vi "ROI_to_INP.vi"(8 "error in (no error)":errorcluster, 9 "Show Message":bool, 10 "ROI Values":T1) -> (0 "error out":errorcluster)   [LabVIEW 2015]
uses:
  <vilib>/Utility/config.llb/Write Key (String).vi
  <vilib>/Utility/config.llb/Write Key (I32).vi
  <vilib>/Utility/config.llb/NI_LVConfig.lvlib
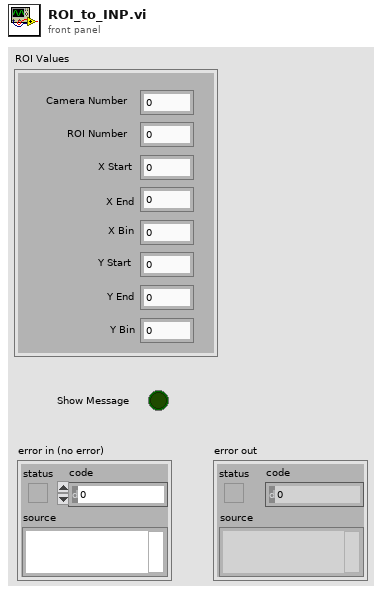
[diagram p1: front panel]
types:
  T1 = cluster{"Camera Number":i32, "ROI Number":i32, "X Start":i32, "X End":i32, "X Bin":i32, "Y Start":i32, "Y End":i32, "Y Bin":i32}
  T2 = typedef "NI_LVConfig.lvlib/Config Data RefNum.ctl" = refnum<k1>
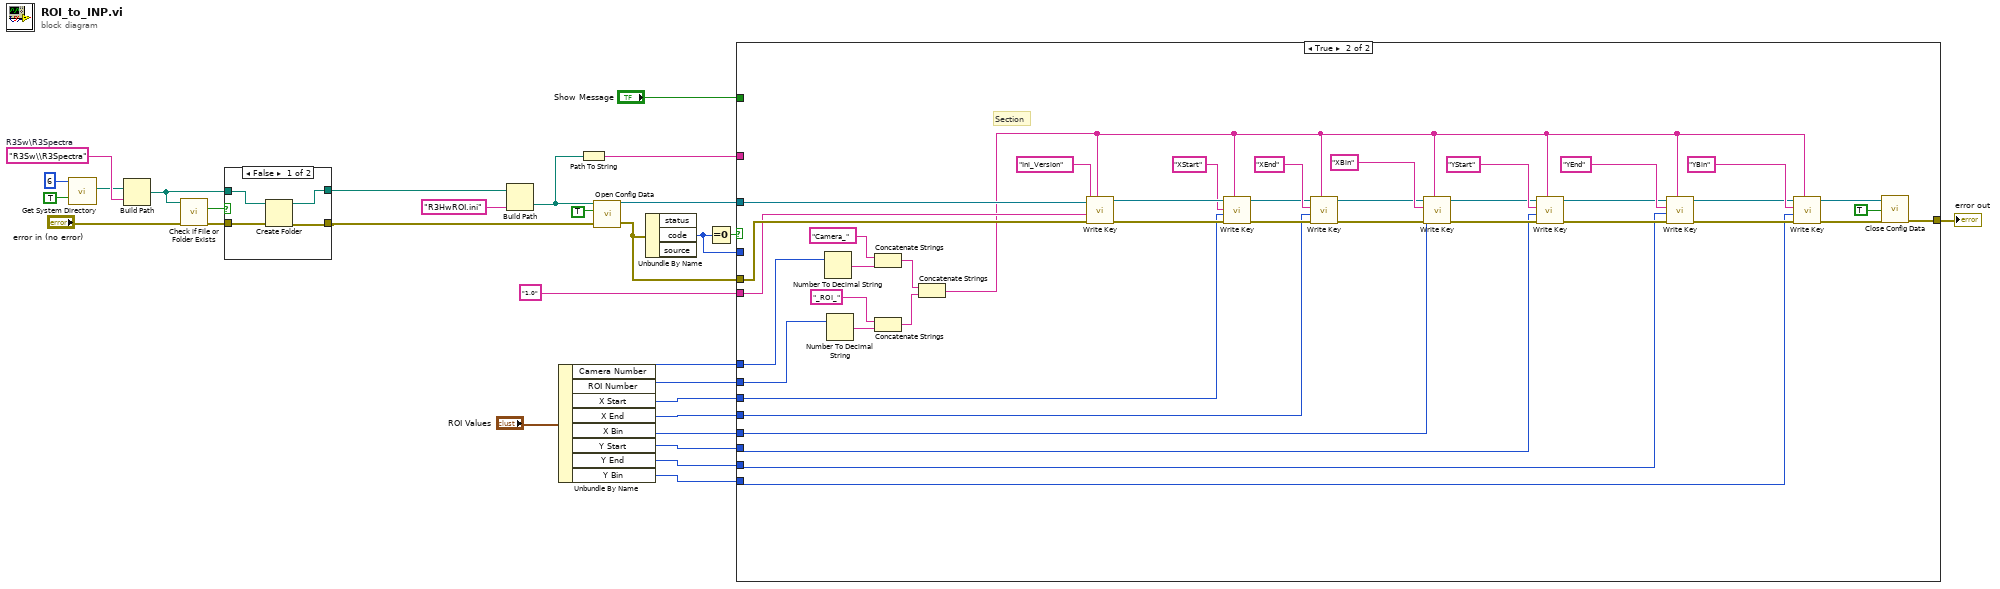
[diagram p0: block diagram]
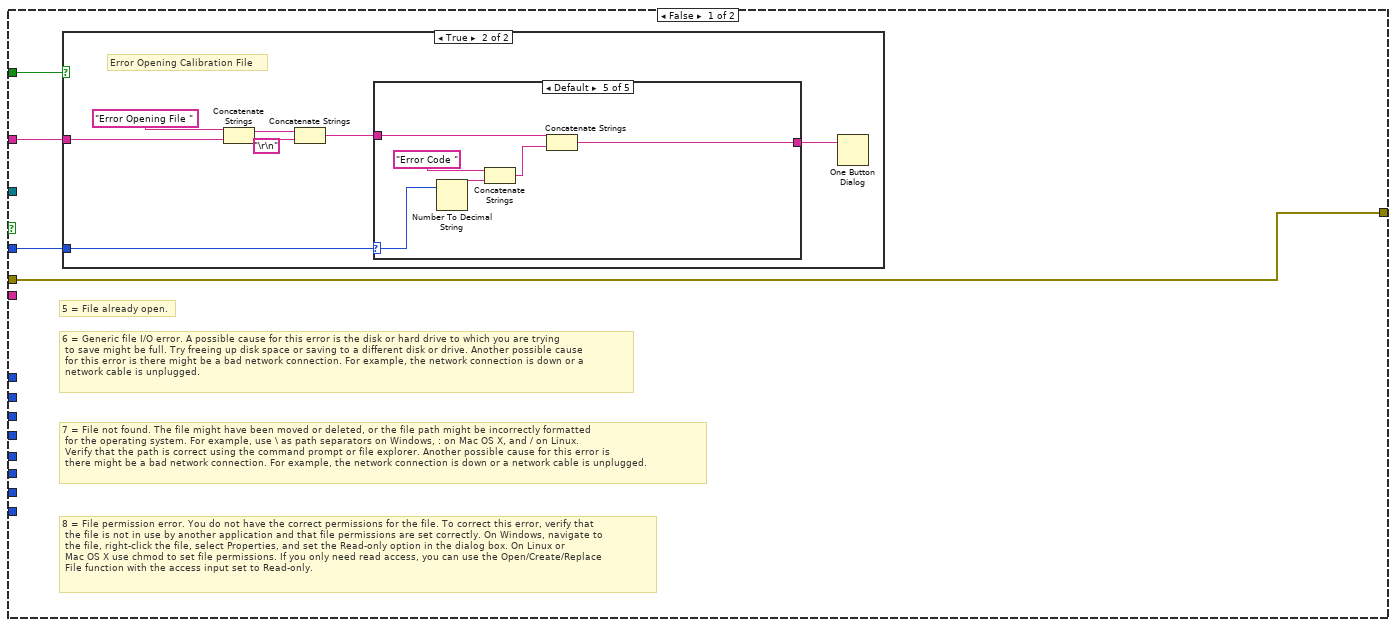
[diagram p3: hidden frame]
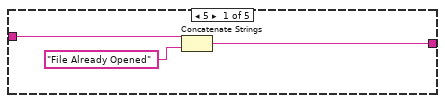
[diagram p5: hidden frame]
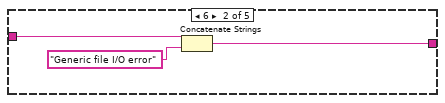
[diagram p6: hidden frame]
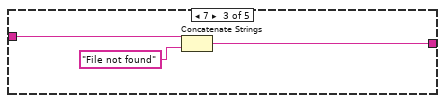
[diagram p7: hidden frame]
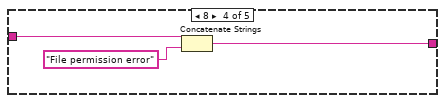
[diagram p8: hidden frame]
diagram:
  w6 = "R3Sw\\R3Spectra"  # R3Sw\R3Spectra
  n1 = call <vilib>:"Get System Directory.vi"("create directory if not found? (F)"=TRUE, "system directory type"=6) -> ("system directory"=w5:path)  [unwired: 9 in]
  n2 = Build Path(base path=w5, name or relative path=w6) -> (appended path=w4:path)
  n3 = call <vilib>:"Check if File or Folder Exists.vi"("error in (no error)"="error in (no error)", "path"=w4) -> ("error out"=w9:errorcluster, "file or folder exists?"=w10:bool)  [unwired: 7 in, 1 out]
  n4 = case shown="False" w10 {
    tunnel: w9 -> [w32 w35]
    tunnel: [w31 w35] -> w2
    tunnel: w4 -> [w33 w34]
    tunnel: [w30 w34] -> w1
    frame False {
      n5 = Create Folder(path (use dialog)=w33, error in=w32) -> (created path=w30:path, error out=w31:errorcluster)  [unwired: 1 in, 1 out]
    }
    frame True {
    }
  }
  n6 = Build Path(base path=w1, name or relative path="R3HwROI.ini") -> (appended path=w16:path)
  n7 = Unbundle By Name("ROI Values") -> ("Camera Number"=w12:i32, "X Start"=w13:i32, "X End"=w22:i32, "X Bin"=w21:i32, "Y Start"=w20:i32, "Y End"=w19:i32, "Y Bin"=w18:i32)  [unwired: 1 out]
  n8 = Path To String(path=w16) -> (string=w15:string)
  n9 = call <vilib>:"Open Config Data.vi"("error in (no error)"=w2, "create file if necessary (T)"=TRUE, "configuration file path"=w16) -> ("error out"=w26:errorcluster, "refnum"=w27:T2)  [unwired: 6 in, 1 out]
  n10 = Unbundle By Name(w26) -> ("code"=w25:i32)  [unwired: 2 out]
  n11 = Equal To 0?(x=w25) -> (x = 0?=w28:bool)
  n12 = case shown="True" w28 {
    tunnel: w27 -> [_ w104]
    tunnel: w26 -> [w37 w103]
    tunnel: w25 -> [w38 _]
    tunnel: w15 -> [w39 _]
    tunnel: [w37 w102] -> w24
    tunnel: w12 -> [_ w100]
    tunnel: "1.0" -> [_ w101]
    tunnel: w13 -> [_ w73]
    tunnel: w22 -> [_ w71]
    tunnel: w21 -> [_ w72]
    tunnel: w20 -> [_ w68]
    tunnel: w19 -> [_ w70]
    tunnel: w18 -> [_ w69]
    tunnel: w12 -> [_ w95]
    tunnel: "Show Message" -> [w36 _]
    frame False {
      # "8 = File permission error. You do not have the correct permissions for the file. To correct this error, verify that\n the file is not in use by another application and that file permissions are set correctly. On Windows, navigate to\n the file, right-click the file, select Properties, and set the Read-only option in the dialog box. On Linux or\n Mac OS X use chmod to set file permissions. If you only need read access, you can use the Open/Create/Replace\n File function with the access input set to Read-only."
      # "7 = File not found. The file might have been moved or deleted, or the file path might be incorrectly formatted\n for the operating system. For example, use \\ as path separators on Windows, : on Mac OS X, and / on Linux.\n Verify that the path is correct using the command prompt or file explorer. Another possible cause for this error is\n there might be a bad network connection. For example, the network connection is down or a network cable is unplugged."
      # "6 = Generic file I/O error. A possible cause for this error is the disk or hard drive to which you are trying\n to save might be full. Try freeing up disk space or saving to a different disk or drive. Another possible cause\n for this error is there might be a bad network connection. For example, the network connection is down or a\n network cable is unplugged."
      # "5 = File already open."
      n13 = case shown="True" w36 {
        tunnel: w39 -> [_ w46]
        tunnel: w38 -> [_ w42]
        frame False {
        }
        frame True {
          # "Error Opening Calibration File"
          n14 = Concatenate Strings("Error Opening File ", w46) -> (w43:string)
          n15 = Concatenate Strings(w43, "\r\n") -> (w41:string)
          n16 = case shown="Default" w42 {
            selector: w42 -> [_ _ _ _ w62]
            tunnel: w41 -> [w48 w51 w54 w57 w64]
            tunnel: [w47 w50 w53 w56 w63] -> w40
            frame 5 {
              n17 = Concatenate Strings(w48, "File Already Opened") -> (w47:string)
            }
            frame 6 {
              n18 = Concatenate Strings(w51, "Generic file I/O error") -> (w50:string)
            }
            frame 7 {
              n19 = Concatenate Strings(w54, "File not found") -> (w53:string)
            }
            frame 8 {
              n20 = Concatenate Strings(w57, "File permission error") -> (w56:string)
            }
            frame Default {
              n21 = Number To Decimal String(number=w62) -> (decimal integer string=w61:string)  [unwired: 1 in]
              n22 = Concatenate Strings("Error Code ", w61) -> (w59:string)
              n23 = Concatenate Strings(w64, w59) -> (w63:string)
            }
          }
          n24 = One Button Dialog(message=w40) -> ()  [unwired: 1 in, 1 out]
        }
      }
    }
    frame True {
      # "Section"
      n25 = Number To Decimal String(number=w95) -> (decimal integer string=w96:string)  [unwired: 1 in]
      n26 = Number To Decimal String(number=w100) -> (decimal integer string=w99:string)  [unwired: 1 in]
      n27 = Concatenate Strings("Camera_", w96) -> (w94:string)
      n28 = Concatenate Strings("_ROI_", w99) -> (w93:string)
      n29 = Concatenate Strings(w94, w93) -> (w90:string)
      n30 = call-poly <vilib>:"Write Key.vi"("section"=w90, "error in (no error)"=w103, "value"=w101, "key"="Ini_Version", "refnum"=w104) -> ("error out"=w91:errorcluster, "refnum out"=w92:T2)  [unwired: 4 in, 1 out]
      n31 = call-poly <vilib>:"Write Key.vi"("section"=w90, "error in (no error)"=w91, "value"=w73, "key"="XStart", "refnum"=w92) -> ("error out"=w78:errorcluster, "refnum out"=w87:T2)  [unwired: 4 in, 1 out]
      n32 = call-poly <vilib>:"Write Key.vi"("section"=w90, "error in (no error)"=w78, "value"=w71, "key"="XEnd", "refnum"=w87) -> ("error out"=w77:errorcluster, "refnum out"=w85:T2)  [unwired: 4 in, 1 out]
      n33 = call-poly <vilib>:"Write Key.vi"("section"=w90, "error in (no error)"=w77, "value"=w72, "key"="XBin", "refnum"=w85) -> ("error out"=w76:errorcluster, "refnum out"=w83:T2)  [unwired: 4 in, 1 out]
      n34 = call-poly <vilib>:"Write Key.vi"("section"=w90, "error in (no error)"=w76, "value"=w68, "key"="YStart", "refnum"=w83) -> ("error out"=w75:errorcluster, "refnum out"=w81:T2)  [unwired: 4 in, 1 out]
      n35 = call-poly <vilib>:"Write Key.vi"("section"=w90, "error in (no error)"=w75, "value"=w70, "key"="YEnd", "refnum"=w81) -> ("error out"=w74:errorcluster, "refnum out"=w79:T2)  [unwired: 4 in, 1 out]
      n36 = call-poly <vilib>:"Write Key.vi"("section"=w90, "error in (no error)"=w74, "value"=w69, "key"="YBin", "refnum"=w79) -> ("error out"=w66:errorcluster, "refnum out"=w67:T2)  [unwired: 4 in, 1 out]
      n37 = call <vilib>:"Close Config Data.vi"("error in (no error)"=w66, "write file if changed (T)"=TRUE, "refnum"=w67) -> ("error out"=w102:errorcluster)  [unwired: 7 in, 1 out]
    }
  }
  "error out" <- w24
